vi "p2.vi"() -> ()   [LabVIEW 2023, in "d2.lvlib"]
uses:
  d2.lvlib
  AOC/AOC.lvlib
panel:
  in  "Input":string="Game 1: 2 green, 6 blue, 7 red; 12 green, 6 blue, 3 red; 5 red, 18 green, 4 blue\nGame 2: 10 green, 4 red; 2 red; 12 green, 11 red, 1 blue; 1 blue, 11 red, 5 green; 10 red, 9 green, 1 blue\nGame 3: 3 green; 15 red, 7 blue, 1 green; 3 red, 6 blue, 1 green; 14 blue, 13 red, 2 green; 1 green, 6 blue, 6 red; 16 red, 13 blue, 2 green\nGame 4: 5 blue; 8 blue, 7 red; 9 blue, 5 red, 4 green; 4 red, 1 green; 8 red, 6 blue; 2 blue, 4 red, 3 green\nGame 5: 3 blue, 4 red, 10 green; 13 green, 8 blue, 2 red; 2 red, 4 green, 6 blue; 3 blue, 5 green, 2 red; 4 red, 13 blue, 8 green; 9 green, 2 red\nGame 6: 3 red, 2 blue; 6 green, 13 blue; 11 blue, 1 red; 4 green, 3 red, 5 blue\nGame 7: 14 green, 2 red, 5 blue; 4 blue, 8 green; 2 red, 2 green, 9 blue\nGame 8: 10 green, 6 blue; 3 green, 4 red; 7 blue, 7 red, 5 green; 1 red, 11 green; 3 blue, 2 red, 11 green\nGame 9: 4 blue, 1 green, 6 red; 5 red, 5 blue; 1 blue, 7 red; 4 red, 8 blue; 6 red\nGame 10: 3 green, 7 blue, 6 red; 1 red, 5 blue; 6 red; 1 red, 5 green, 6 blue; 5 red, 2 blue; 6 red, 4 blue, 6 green\nGame 11: 8 red, 6 blue, 6 green; 5 blue, 2 red, 5 green; 4 blue, 5 green; 4 blue, 3 red, 8 green\nGame 12: 5 green, 1 red, 7 blue; 1 red, 10 green; 6 red, 3 green, 7 blue; 5 red, 6 blue, 7 green; 3 blue, 4 green; 1 red, 3 blue, 3 green\nGame 13: 11 red, 9 blue, 16 green; 1 red, 3 green, 3 blue; 14 green, 2 red, 7 blue\nGame 14: 4 red, 8 blue, 12 green; 7 blue, 4 red, 2 green; 4 blue, 7 green, 6 red; 3 red, 11 blue, 12 green\nGame 15: 6 red; 3 red, 5 blue; 3 red, 10 blue, 1 green; 2 green, 8 red, 2 blue\nGame 16: 2 green, 4 red, 6 blue; 2 green, 16 blue, 2 red; 13 blue, 7 green, 3 red\nGame 17: 5 blue; 1 blue; 2 red, 2 green, 4 blue; 6 blue, 4 green, 2 red\nGame 18: 3 red; 7 green, 11 red, 6 blue; 6 red, 3 blue, 12 green; 5 red, 3 blue; 7 green, 8 red, 9 blue\nGame 19: 2 green, 13 blue; 11 blue, 16 red, 7 green; 13 blue, 10 green, 8 red; 18 red, 1 green, 14 blue\nGame 20: 10 red, 6 green; 1 blue, 6 red, 15 green; 15 green, 9 red, 3 blue; 3 blue, 11 red, 9 green; 2 blue, 5 red, 10 green\nGame 21: 1 green, 5 red, 8 blue; 4 red, 6 green, 7 blue; 13 blue, 10 green, 6 red; 9 blue, 2 red, 14 green; 16 green, 10 blue, 1 red; 9 blue, 3 red, 11 green\nGame 22: 4 blue; 1 green, 1 red, 16 blue; 15 blue, 1 red\nGame 23: 2 blue, 6 green; 15 green, 2 blue, 10 red; 1 green, 6 blue, 6 red; 8 red, 1 green; 4 green, 3 blue, 10 red; 7 red, 3 blue, 20 green\nGame 24: 1 red, 13 blue, 8 green; 3 blue, 7 red, 8 green; 3 red, 11 green, 12 blue; 7 green, 6 blue, 2 red; 11 blue, 5 red, 10 green; 13 blue, 3 green, 8 red\nGame 25: 4 red, 6 green, 8 blue; 4 red, 10 blue, 9 green; 5 red, 2 blue, 3 green; 2 green, 9 red, 4 blue\nGame 26: 14 red, 4 green, 5 blue; 3 blue, 2 red, 3 green; 1 red, 9 blue, 1 green; 5 green, 15 red, 8 blue; 5 green, 6 red, 6 blue\nGame 27: 1 blue, 1 green, 9 red; 4 green, 1 blue, 1 red; 4 green, 4 red; 5 green, 4 red; 1 green, 1 blue, 8 red; 9 red\nGame 28: 11 red, 3 blue, 19 green; 3 green, 13 red, 5 blue; 8 blue, 16 red, 18 green; 13 red, 5 blue, 7 green; 8 red, 5 green, 4 blue; 16 green, 1 blue, 15 red\nGame 29: 12 red, 15 blue, 1 green; 3 green, 10 red, 5 blue; 4 green, 5 blue, 17 red; 11 red, 2 blue; 6 blue, 3 green, 4 red; 1 blue, 13 red\nGame 30: 2 blue, 2 green, 3 red; 1 green, 4 red; 1 red, 2 blue; 1 green, 1 blue, 2 red\nGame 31: 3 green, 5 blue, 4 red; 3 red, 1 green; 3 blue, 4 red, 3 green; 8 blue, 8 red; 6 blue; 1 green, 6 blue, 1 red\nGame 32: 3 blue, 12 green, 2 red; 13 red, 12 green, 4 blue; 9 green, 1 red; 10 red; 12 green, 9 red; 15 red, 3 blue, 10 green\nGame 33: 1 green, 8 blue; 3 red, 7 green; 4 red, 3 green; 5 red, 9 green\nGame 34: 12 blue, 3 red, 2 green; 12 blue, 12 green, 2 red; 10 blue, 8 green; 3 red, 3 green, 9 blue\nGame 35: 4 red, 4 blue, 6 green; 3 blue, 8 green, 2 red; 5 green, 2 red, 2 blue\nGame 36: 12 blue, 4 red, 5 green; 18 blue, 2 red, 5 green; 2 green, 2 red; 3 red, 9 green, 13 blue; 2 green, 12 blue, 1 red\nGame 37: 8 red, 3 blue; 6 blue, 5 red; 9 red, 10 blue, 3 green; 4 green, 10 red\nGame 38: 1 green, 3 blue, 7 red; 6 blue, 6 green, 9 red; 5 green\nGame 39: 7 red, 1 blue, 1 green; 5 red, 2 blue, 3 green; 9 red, 9 blue; 5 red, 3 green, 1 blue; 1 green, 9 red, 1 blue\nGame 40: 1 blue, 1 green, 3 red; 3 red, 2 green, 2 blue; 5 red, 1 blue, 8 green; 2 green, 4 red, 2 blue; 13 red, 2 green\nGame 41: 17 blue, 5 red, 3 green; 10 green, 4 red, 5 blue; 3 red, 17 blue, 1 green; 11 blue, 10 red, 3 green\nGame 42: 8 blue, 2 green, 7 red; 4 blue, 1 red; 9 red, 2 green, 6 blue; 4 blue, 9 red; 1 green, 9 blue, 8 red; 6 red, 1 green\nGame 43: 1 green, 6 blue, 14 red; 7 green, 1 blue, 8 red; 3 green, 16 red, 7 blue\nGame 44: 5 red, 5 blue; 1 green, 8 red, 9 blue; 6 red, 3 blue\nGame 45: 4 green, 17 red, 14 blue; 14 red, 2 green, 2 blue; 9 blue, 1 green, 8 red\nGame 46: 1 blue, 10 red, 7 green; 3 red, 4 blue; 2 blue, 1 green, 1 red\nGame 47: 8 red, 2 green, 13 blue; 10 red, 9 blue; 4 green, 15 blue, 2 red; 1 blue, 1 green, 16 red\nGame 48: 9 red, 8 green, 1 blue; 10 green, 5 red; 9 red, 3 green, 1 blue; 8 red, 1 green\nGame 49: 11 blue, 18 green, 1 red; 13 red, 9 blue; 17 green, 18 red, 6 blue\nGame 50: 2 green, 10 red, 6 blue; 6 red, 6 blue, 7 green; 7 red, 5 green, 3 blue; 5 green, 2 red, 1 blue\nGame 51: 1 blue, 9 green, 7 red; 2 blue, 11 red, 10 green; 1 blue, 9 green, 12 red; 10 red, 5 green, 3 blue; 9 green, 3 blue, 14 red\nGame 52: 4 green; 6 blue; 4 green, 7 blue; 1 blue; 1 red, 8 green, 1 blue\nGame 53: 6 green, 3 blue, 13 red; 3 blue, 2 green, 16 red; 13 red, 9 green, 2 blue; 1 red, 1 blue, 7 green\nGame 54: 1 green, 4 blue, 10 red; 2 red, 6 blue; 2 blue, 5 red; 3 blue, 7 red, 1 green\nGame 55: 17 red; 18 red, 3 blue, 4 green; 5 blue, 14 red, 1 green; 4 green, 5 blue, 4 red; 2 green, 18 red\nGame 56: 14 green, 2 red, 18 blue; 8 green, 12 blue, 2 red; 1 red, 13 blue, 12 green\nGame 57: 2 green, 4 blue, 12 red; 1 green, 3 red, 4 blue; 4 green, 2 red, 3 blue; 3 green, 6 red; 3 red, 3 blue, 3 green\nGame 58: 2 blue, 5 red, 2 green; 6 red, 6 green; 8 red, 11 green, 2 blue; 9 green, 1 blue, 11 red; 2 blue, 17 green, 11 red; 7 red, 8 green, 2 blue\nGame 59: 4 blue, 1 red, 16 green; 2 blue, 5 green, 1 red; 2 green, 6 blue; 3 blue, 10 green; 14 green, 6 blue; 1 red, 11 green\nGame 60: 4 red, 1 blue, 5 green; 2 green, 6 blue; 1 red, 17 green; 2 red, 11 blue, 14 green; 2 red, 8 blue, 14 green\nGame 61: 6 red, 7 blue, 1 green; 2 red, 10 green, 16 blue; 14 blue, 10 green, 7 red; 12 red, 15 blue, 3 green; 5 blue, 1 red\nGame 62: 9 blue, 4 red; 1 green, 2 blue, 4 red; 8 red, 9 blue; 6 red, 15 blue; 7 blue, 10 red\nGame 63: 8 green, 2 red, 4 blue; 2 red, 1 green, 3 blue; 1 red, 3 green; 2 blue, 9 green\nGame 64: 4 green, 13 red; 2 red, 6 green, 2 blue; 4 red, 6 green, 2 blue; 6 red, 2 blue; 5 red, 9 green; 3 red, 1 blue, 10 green\nGame 65: 8 blue, 3 red, 3 green; 6 red, 8 green; 6 blue, 7 green, 7 red\nGame 66: 6 red, 2 blue, 2 green; 15 green, 11 red, 1 blue; 1 red, 2 blue, 10 green; 2 blue, 17 green; 12 green, 2 blue, 4 red; 16 green, 10 red, 3 blue\nGame 67: 1 green, 2 red, 12 blue; 2 red, 3 blue, 3 green; 8 blue, 4 green, 1 red; 12 blue, 2 red, 4 green; 2 red, 10 blue\nGame 68: 6 red, 4 green, 16 blue; 9 red, 7 green, 11 blue; 7 blue, 16 green, 15 red; 2 red, 2 green; 16 red; 13 red, 15 green, 2 blue\nGame 69: 14 red, 3 blue, 14 green; 4 blue, 18 green, 2 red; 4 green, 9 blue, 7 red; 15 green, 9 blue, 10 red\nGame 70: 2 green, 5 red, 12 blue; 3 green, 5 red, 4 blue; 5 blue, 4 red; 6 red, 11 blue; 5 red, 2 blue; 5 blue, 1 green, 4 red\nGame 71: 3 green, 3 red; 6 green, 11 blue, 2 red; 6 red, 4 blue\nGame 72: 9 blue, 4 green, 4 red; 5 blue, 5 red, 3 green; 9 blue, 11 green, 3 red\nGame 73: 1 blue, 13 red; 12 red; 5 red, 1 green, 6 blue; 5 blue, 7 red; 8 red, 9 blue\nGame 74: 7 green, 17 red, 3 blue; 15 red, 2 green; 5 red, 3 blue, 1 green; 19 red, 1 blue; 3 red, 1 blue, 6 green; 7 red, 3 blue, 1 green\nGame 75: 11 blue, 9 green, 4 red; 5 green, 2 red, 16 blue; 13 blue, 2 red; 3 red, 18 blue, 1 green\nGame 76: 5 green, 13 red, 10 blue; 5 red, 11 green; 1 red, 5 green, 8 blue; 4 red, 14 green; 7 blue, 12 green, 2 red\nGame 77: 5 blue, 2 green, 3 red; 2 red; 1 green, 6 blue; 5 blue, 1 red\nGame 78: 9 red, 7 green; 10 red, 2 blue, 6 green; 13 red, 3 blue, 15 green; 9 blue, 10 green, 2 red; 1 blue, 4 red, 12 green\nGame 79: 4 red, 3 green; 3 blue, 10 green, 4 red; 1 red, 12 green, 7 blue; 5 blue, 3 green, 6 red; 10 green, 1 blue, 5 red; 5 green, 5 red\nGame 80: 3 blue, 18 green; 5 blue, 11 green, 3 red; 2 blue, 13 green, 7 red; 4 red, 1 blue, 8 green\nGame 81: 9 green, 18 blue, 10 red; 6 red, 5 green, 13 blue; 8 red, 4 blue, 7 green\nGame 82: 9 green, 2 red, 2 blue; 7 green, 2 red, 1 blue; 2 green, 2 red, 2 blue; 2 red, 14 green, 1 blue\nGame 83: 10 red, 7 green, 3 blue; 4 green, 12 red, 12 blue; 13 blue, 1 green, 8 red\nGame 84: 10 green, 3 blue; 8 green, 2 red; 3 blue, 5 green; 3 blue, 1 green; 5 blue, 7 green, 1 red; 8 green, 5 blue, 2 red\nGame 85: 6 blue, 4 green, 5 red; 11 green, 1 blue, 13 red; 11 green, 1 red; 6 green, 2 red; 1 blue, 5 green, 4 red\nGame 86: 1 blue, 10 red; 2 blue, 5 red; 1 red, 2 blue, 2 green\nGame 87: 11 green, 13 red, 6 blue; 8 blue, 2 red, 6 green; 10 blue, 11 red, 1 green; 16 green, 16 blue, 6 red; 6 green, 12 red, 3 blue\nGame 88: 15 green, 4 red, 2 blue; 6 red, 13 green, 4 blue; 3 green, 17 red, 4 blue; 4 blue, 14 green\nGame 89: 6 green, 12 red, 7 blue; 3 blue, 6 green, 7 red; 6 green, 13 red, 5 blue; 6 red, 7 green\nGame 90: 19 blue, 19 red; 6 blue, 12 red, 6 green; 2 green, 7 blue, 17 red; 3 green, 9 blue, 7 red; 8 red, 7 green, 18 blue\nGame 91: 3 red, 1 green; 14 red, 2 blue, 2 green; 7 red, 3 blue; 1 blue, 6 red\nGame 92: 2 green, 16 red, 15 blue; 3 green, 3 blue, 11 red; 7 blue, 6 red; 7 blue, 13 red\nGame 93: 1 red, 1 blue, 9 green; 12 green, 3 red, 4 blue; 3 green, 3 red, 7 blue\nGame 94: 12 green, 5 red, 9 blue; 3 blue, 3 green, 2 red; 5 green, 2 blue; 5 green, 7 red, 10 blue; 7 red, 10 blue, 10 green\nGame 95: 3 blue, 15 red, 10 green; 3 blue, 16 red; 1 blue, 13 green, 6 red\nGame 96: 11 blue, 2 green, 5 red; 2 green, 10 red, 15 blue; 11 blue, 19 red, 8 green\nGame 97: 7 green, 2 red, 1 blue; 5 red, 3 blue, 12 green; 4 blue, 2 green, 3 red\nGame 98: 2 green, 5 blue, 9 red; 4 green, 9 blue, 8 red; 7 green, 11 blue, 7 red\nGame 99: 2 green, 15 blue, 2 red; 2 red, 6 green, 12 blue; 11 green, 18 blue, 2 red; 3 red, 9 blue, 3 green; 18 blue\nGame 100: 13 red, 2 green; 15 red, 1 green; 4 green, 1 blue; 11 red, 5 green; 3 green, 8 red\n"
  in  "Example":string="Game 1: 3 blue, 4 red; 1 red, 2 green, 6 blue; 2 green\nGame 2: 1 blue, 2 green; 3 green, 4 blue, 1 red; 1 green, 1 blue\nGame 3: 8 green, 6 blue, 20 red; 5 blue, 4 red, 13 green; 5 green, 1 red\nGame 4: 1 green, 3 red, 6 blue; 3 green, 6 red; 3 green, 15 blue, 14 red\nGame 5: 6 red, 1 blue, 3 green; 2 blue, 1 red, 2 green"
  in  "Example":bool
  out "Answer":i64=10624
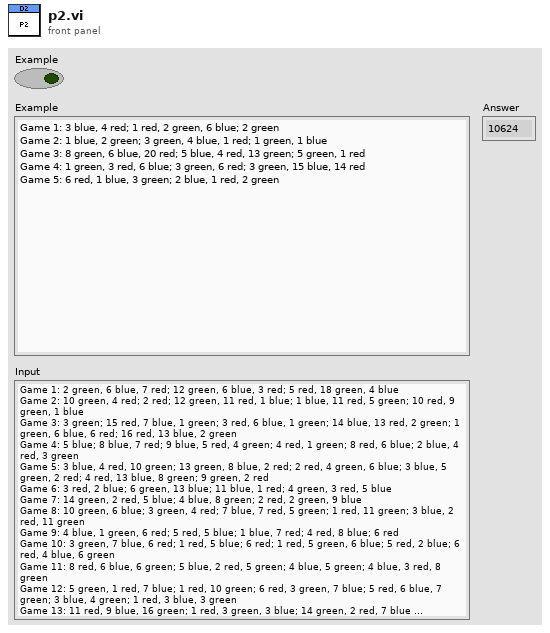
[diagram p1: front panel]
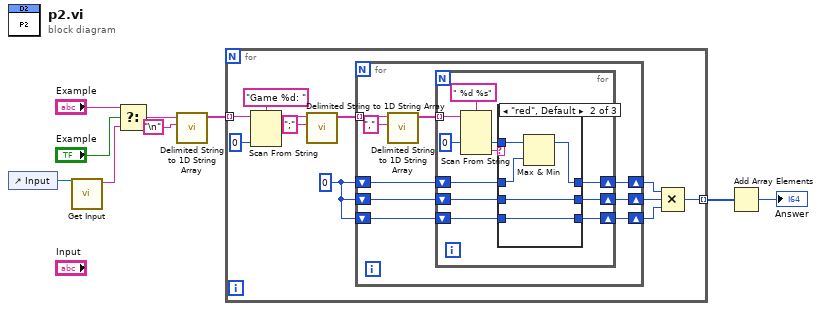
[diagram p0: block diagram]
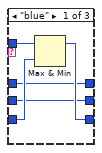
[diagram p2: hidden frame]
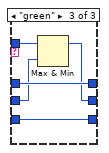
[diagram p3: hidden frame]
diagram:
  n1 = control-ref of="Input"() -> (w1:refnum<vi>)
  n2 = call "Get Input.vi"("Input ref"=w1) -> ("Input"=w9:string)  [unwired: 10 in]
  n3 = Select(t="Example", s="Example", f=w9) -> (s? t:f=w8:string)
  n4 = call <vilib>:"Delimited String to 1D String Array.vi"("delimiter"="\n", "delimited string"=w8) -> ("string array"=w6:string[])  [unwired: 9 in]
  n5 = for {
    tunnel: w6 -> [w20] mode=indexing
    tunnel: [w10] -> w3 mode=indexing
    w14 = i64 0 ("y")
    n6 = Scan From String(format string="Game %d: ", input string=w20, default 1=i64 0 ("default value 1")) -> (remaining string=w15:string)  [unwired: 3 in, 2 out]
    n7 = call <vilib>:"Delimited String to 1D String Array.vi"("delimiter"=";", "delimited string"=w15) -> ("string array"=w17:string[])  [unwired: 9 in]
    n8 = for {
      tunnel: w17 -> [w29] mode=indexing
      shift-right: [w23] -> w13
      shift-left: w14 -> [w26]
      shift-right: [w22] -> w12
      shift-left: w14 -> [w25]
      shift-right: [w21] -> w11
      shift-left: w14 -> [w24]
      n9 = call <vilib>:"Delimited String to 1D String Array.vi"("delimiter"=",", "delimited string"=w29) -> ("string array"=w27:string[])  [unwired: 9 in]
      n10 = for {
        tunnel: w27 -> [w40] mode=indexing
        shift-right: [w31] -> w23
        shift-left: w26 -> [w32]
        shift-right: [w33] -> w22
        shift-left: w25 -> [w34]
        shift-right: [w35] -> w21
        shift-left: w24 -> [w36]
        n11 = Scan From String(format string=" %d %s", input string=w40, default 1=i64 0 ("default value 1")) -> (output 1=w37:i64, output 2=w38:string)  [unwired: 3 in, 3 out]
        n12 = case shown="\"red\", Default" w38 {
          tunnel: w36 -> [w44 w46 w54]
          tunnel: w37 -> [w45 w50 w55]
          tunnel: [w43 w46 w54] -> w35
          tunnel: w34 -> [w42 w49 w51]
          tunnel: [w42 w49 w52] -> w33
          tunnel: w32 -> [w41 w48 w53]
          tunnel: [w41 w47 w53] -> w31
          frame "blue" {
            n13 = Max & Min(x=w45, y=w44) -> (max(x,y)=w43:i64)  [unwired: 1 out]
          }
          frame "red", Default {
            n14 = Max & Min(x=w50, y=w48) -> (max(x,y)=w47:i64)  [unwired: 1 out]
          }
          frame "green" {
            n15 = Max & Min(x=w55, y=w51) -> (max(x,y)=w52:i64)  [unwired: 1 out]
          }
        }
      }
    }
    n16 = Compound Arithmetic op=MULTIPLY(w13, w12, w11) -> (w10:i64)
  }
  n17 = Add Array Elements(numeric array=w3) -> (sum=→"Answer":i64)
